vi "getGain.vi"(8 "error in":errorcluster, 10 "CtrlV":dbl, 11 "APD":T1) -> (0 "error out":errorcluster, 2 "gain":dbl)   [LabVIEW 2020]
uses:
  APD.ctl
  <vilib>/gmath/NI_Gmath.lvlib
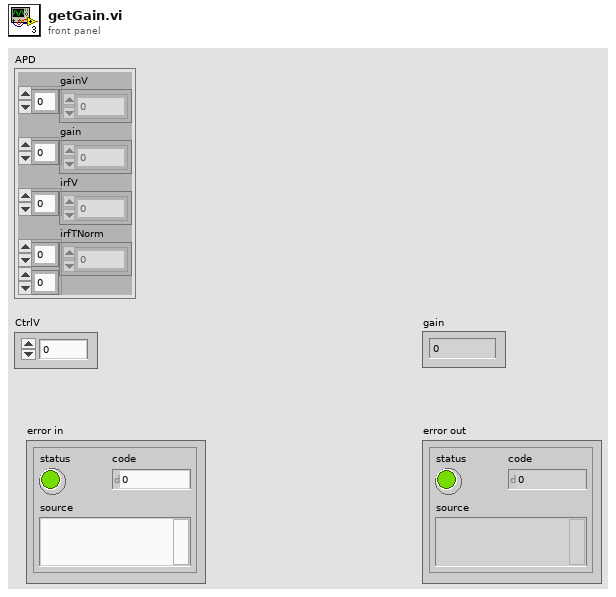
[diagram p1: front panel]
types:
  T1 = typedef "APD.ctl" = cluster{"gainV":dbl[], "gain":dbl[], "irfV":dbl[], "irfTNorm":dbl[][]}
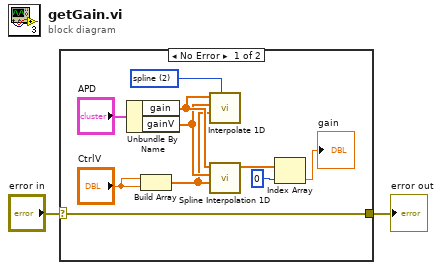
[diagram p0: block diagram]
diagram:
  n1 = case shown="No Error" "error in" {
    selector: "error in" -> [w3 w13]
    tunnel: [w3 w13] -> w1
    frame No Error {
      w10 = 2 items=["nearest", "linear", "spline", "cubic Hermite", "Lagrange"] ("method")
      n2 = Unbundle By Name("APD") -> ("gain"=w7:dbl[], "gainV"=w6:dbl[])
      n3 = Build Array("CtrlV", "CtrlV") -> (w5:dbl[])
      n4 = call <vilib>:"Interpolate 1D.vi"("method"=w10, "xi"=w5, "X"=w6, "Y"=w7) -> ()  [unwired: 5 in, 3 out]
      n5 = call <vilib>:"Spline Interpolation 1D.vi"("xi"=w5, "X"=w6, "Y"=w7) -> ("yi"=w4:dbl[])  [unwired: 6 in, 2 out]
      n6 = Index Array(array=w4, index=0) -> (element=→"gain":dbl)
    }
    frame Error {
    }
  }
  "error out" <- w1
